vi "Check Equal Contents.vi"(8 "error in (no error)":errorcluster, 10 "Pointer y":refnum<class "Pointer.lvclass">, 11 "Pointer x":refnum<class "Pointer.lvclass">) -> (0 "error out":errorcluster, 1 "equal contents?":bool, 2 "Pointer y":refnum<class "Pointer.lvclass">, 3 "Pointer x":refnum<class "Pointer.lvclass">)   [LabVIEW 2027, in "Memory Manager.lvlib" / "Pointer.lvclass"]
doc: "Reads and compares the data from both <b>Pointers</b>. If the size and contents are equal, this function returns TRUE."
uses:
  Pointer.lvclass
  Read 1D U8.vi
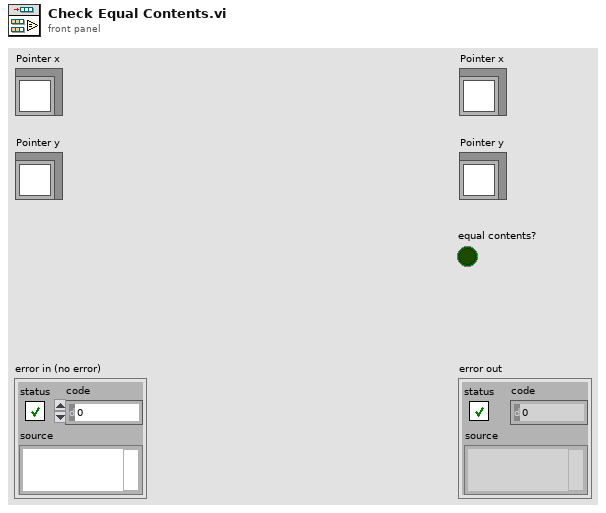
[diagram p1: front panel]
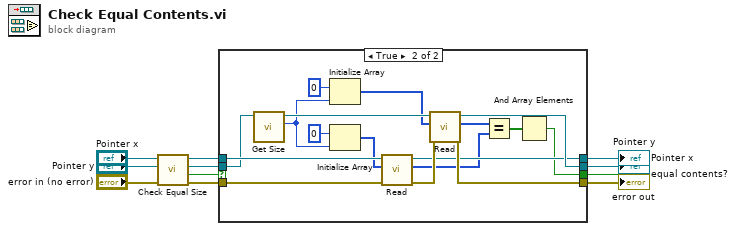
[diagram p0: block diagram]
diagram:
  n1 = call "Check Equal Size.vi"("error in (no error)"="error in (no error)", "Pointer y"="Pointer y", "Pointer x"="Pointer x") -> ("error out"=w5:errorcluster, "equal size?"=w8:bool, "Pointer y"=w6:refnum<class "Pointer.lvclass">, "Pointer x"=w7:refnum<class "Pointer.lvclass">)  [unwired: 5 in]
  n2 = case shown="True" w8 {
    selector: w8 -> [w12 _]
    tunnel: w7 -> [w15 w30]
    tunnel: w6 -> [w14 w25]
    tunnel: w5 -> [w13 w26]
    tunnel: [w15 w19] -> w4
    tunnel: [w14 w21] -> w3
    tunnel: [w13 w27] -> w2
    tunnel: [w12 w17] -> w1
    frame False {
    }
    frame True {
      n3 = call "Get Size.vi"("Pointer in"=w25) -> ("size"=w23:u64, "Pointer out"=w24:refnum<class "Pointer.lvclass">)  [unwired: 9 in]
      n4 = Initialize Array(u8 0 ("element"), w23) -> (w16:u8[])
      n5 = Initialize Array(u8 0 ("element"), w23) -> (w29:u8[])
      n6 = call-poly "Read.vi"("error in (no error)"=w26, "buffer in"=w29, "Pointer in"=w30) -> ("error out"=w28:errorcluster, "buffer out"=w18:u8[], "Pointer out"=w19:refnum<class "Pointer.lvclass">)  [unwired: 5 in, 1 out]
      n7 = call-poly "Read.vi"("error in (no error)"=w28, "buffer in"=w16, "Pointer in"=w24) -> ("error out"=w27:errorcluster, "buffer out"=w22:u8[], "Pointer out"=w21:refnum<class "Pointer.lvclass">)  [unwired: 5 in, 1 out]
      n8 = Equal?(x=w22, y=w18) -> (x = y?=w20:bool[])
      n9 = And Array Elements(Boolean array=w20) -> (logical AND=w17:bool)
    }
  }
  "error out" <- w2
  "Pointer x" <- w4
  "Pointer y" <- w3
  "equal contents?" <- w1
